vi "G#Object_GetClassPath.vi"(0 "reference in":refnum<class "G#RemoteProxy.lvclass">, 5 "error in (no error)":errorcluster) -> (14 "reference out":refnum<class "G#RemoteProxy.lvclass">, 15 "class path":path, 19 "error out":errorcluster)   [LabVIEW 2020, in "G#RemoteProxy.lvclass"]
doc: "Returns the path to the lvclass file."
uses:
  <vilib>/addons/_AddQ/G#Debugger/G#RemoteProxy/G#RemoteProxy.lvclass
  <vilib>/addons/_AddQ/G#Debugger/G#RemoteProxy/G#RemoteProxy.lvclass/G#RemoteProxy.ctl
  <vilib>/addons/_AddQ/G#Object/G#Object.lvclass
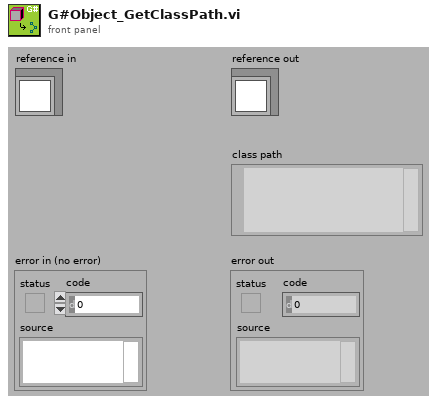
[diagram p1: front panel]
types:
  T1 = typedef "G#RemoteProxy.lvclass/ObjectAttributesProxy.ctl" = cluster{"class hierarchy":T2[], "class name":string, "lvlib hierarchy":string[], "full class name":string, "id":u32, "owner":string, "RemoteRef":refnum<class "G#Object.lvclass">, "object name":string, "attributes":variant[], "connection ID":refnum<k5>, "address":u32, "occurrence":refnum<k4>, "ProxyClassRef":refnum<class "G#RemoteProxy.lvclass">, "InMemory?":bool, "ToString":string}
  T2 = typedef "G#Object.lvclass/G#Object_ClassHierarchy.ctl" = cluster{"ClassName":string, "FullClassName":string, "ClassPath":path, "IsLeaf":bool}
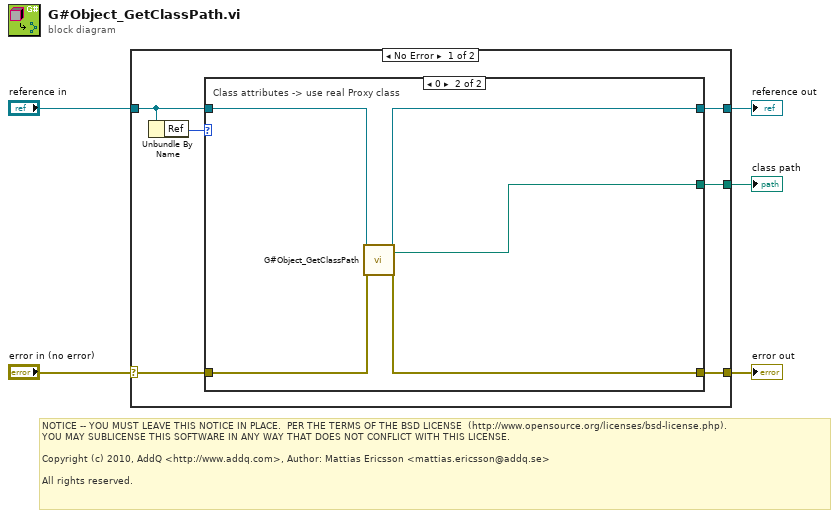
[diagram p0: block diagram]
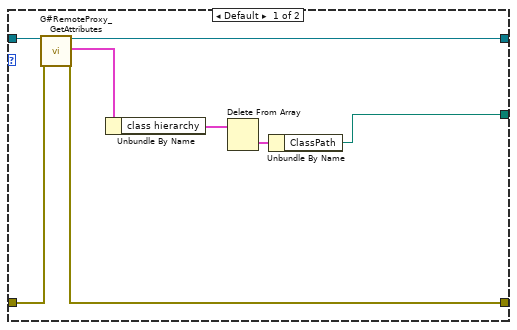
[diagram p2: hidden frame]
diagram:
  # "NOTICE -- YOU MUST LEAVE THIS NOTICE IN PLACE.  PER THE TERMS OF THE BSD LICENSE  (http://www.opensource.org/licenses/bsd-license.php).\nYOU MAY SUBLICENSE THIS SOFTWARE IN ANY WAY THAT DOES NOT CONFLICT WITH THIS LICENSE.\n\nCopyright (c) 2010, AddQ <http://www.addq.com>, Author: Mattias Ericsson <mattias.ericsson@addq.se>\n\nAll rights reserved."
  n1 = case shown="No Error" "error in (no error)" {
    selector: "error in (no error)" -> [w10 w26]
    tunnel: [w9 w26] -> w4
    tunnel: [w11 w25] -> w2
    tunnel: "reference in" -> [w7 w25]
    tunnel: [w8 _] -> w1
    frame No Error {
      n2 = Unbundle By Name(w7) -> ("Ref"=w6:u32)
      n3 = case shown="0" w6 {
        tunnel: [w19 w20] -> w11
        tunnel: w10 -> [w18 w23]
        tunnel: [w17 w22] -> w9
        tunnel: [w13 w21] -> w8
        tunnel: w7 -> [w12 w24]
        frame Default {
          n4 = call <vilib>:"G#RemoteProxy_GetAttributes.vi"("reference in"=w12, "error in (no error)"=w18) -> ("reference out"=w19:refnum<class "G#RemoteProxy.lvclass">, "attributes"=w16:T1, "error out"=w17:errorcluster)  [unwired: 14 in, 1 out]
          n5 = Unbundle By Name(w16) -> ("class hierarchy"=w15:T2[])
          n6 = Delete From Array(array=w15) -> (deleted portion=w14:T2)  [unwired: 2 in, 1 out]
          n7 = Unbundle By Name(w14) -> ("ClassPath"=w13:path)
        }
        frame 0 {
          # "Class attributes -> use real Proxy class"
          n8 = call-parent "G#Object_GetClassPath.vi"("reference in"=w24, "error in (no error)"=w23) -> ("reference out"=w20:refnum<class "G#RemoteProxy.lvclass">, "class path"=w21:path, "error out"=w22:errorcluster)  [unwired: 15 in]
        }
      }
    }
    frame Error {
    }
  }
  "error out" <- w4
  "reference out" <- w2
  "class path" <- w1
